vi "AcPwrRemovedotInstrument.vi"(11 "ModuleList":string[](array[string])=["AcPwr.PPS", "AcPwr.Chroma"]) -> (2 "BeforeMatch-RedundantEntries":string[](array[string]), 3 "Before Match":string[](array[string]), 5 "AfterMatch":string[](array[string]))   [LabVIEW 2018]
doc: "This VI strips out the [.xxx] from the \"yyy.xxx\". Where xxx is the type name and yyy is the module name. This function is helpful when using multiple types of the same module."
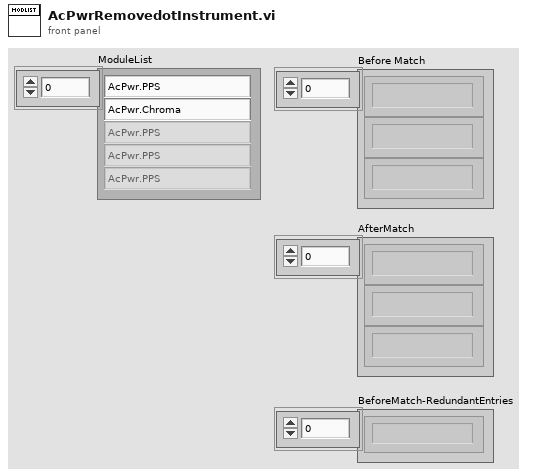
[diagram p1: front panel]
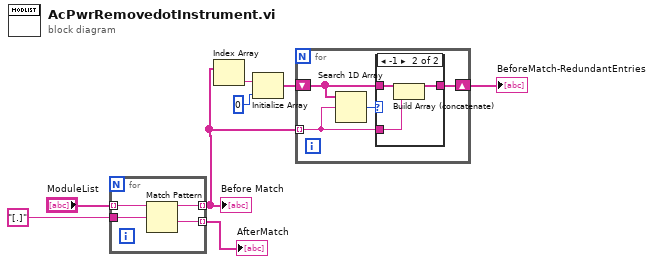
[diagram p0: block diagram]
diagram:
  n1 = for {
    tunnel: "ModuleList" -> [w12] mode=indexing
    tunnel: [w11] -> w1 mode=indexing
    tunnel: [w10] -> w3 mode=indexing
    tunnel: "[.]" ("regular expression") -> [w9]
    n2 = Match Pattern(string=w12, regular expression=w9) -> (before substring=w11:string, after substring=w10:string)  [unwired: 1 in, 2 out]
  }
  "Before Match" <- w1
  "AfterMatch" <- w3
  n3 = Index Array(array=w1) -> (element=w4:string)  [unwired: 1 in]
  n4 = Initialize Array(w4, 0 ("Dimension Size")) -> (w5:string[])
  n5 = for {
    tunnel: w1 -> [w15] mode=indexing
    shift-right: [w14] -> w2
    shift-left: w5 -> [w13]
    n6 = Search 1D Array(1D array=w13, element=w15) -> (index of element=w16:i32)  [unwired: 1 in]
    n7 = case shown="-1" w16 {
      tunnel: w15 -> [_ w20]
      tunnel: [w17 w18] -> w14
      tunnel: w13 -> [w17 w19]
      frame Default {
      }
      frame -1 {
        n8 = Build Array (concatenate)(w19, w20) -> (w18:string[])
      }
    }
  }
  "BeforeMatch-RedundantEntries" <- w2
